vi "pwd.vi"() -> (3 "array of strings":string[](array[string]))   [LabVIEW 2017]
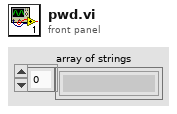
[diagram p1: front panel]
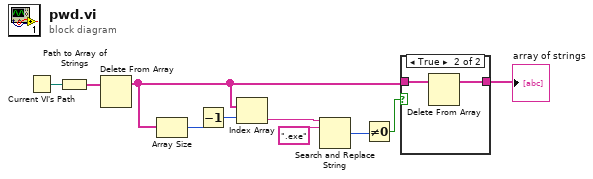
[diagram p0: block diagram]
diagram:
  n1 = Current VI's Path() -> (path=w2:path)
  n2 = Path to Array of Strings(0:w2) -> (2:w1:string[])  [unwired: 1 out]
  n3 = Delete From Array(array=w1) -> (array with subset deleted=w9:string[])  [unwired: 2 in, 1 out]
  n4 = Array Size(array=w9) -> (size(s)=w3:i32)
  n5 = Decrement(x=w3) -> (x-1=w4:i32)
  n6 = Index Array(array=w9, index=w4) -> (element=w5:string)
  n7 = Search and Replace String(input string=w5, search string=".exe") -> (number of replacements=w7:i32)  [unwired: 6 in, 3 out]
  n8 = Not Equal To 0?(x=w7) -> (x != 0?=w8:bool)
  n9 = case shown="True" w8 {
    tunnel: w9 -> [w11 w13]
    tunnel: [w11 w12] -> w10
    frame False {
    }
    frame True {
      n10 = Delete From Array(array=w13) -> (array with subset deleted=w12:string[])  [unwired: 2 in, 1 out]
    }
  }
  "array of strings" <- w10
